vi "4461.Create.Sample Clock.vi"(8 "error in (no error)":errorcluster, 11 "LockinDAQ":refnum<class "LockinDAQ.lvclass">) -> (0 "error out":errorcluster, 3 "LockinDAQ out":refnum<class "LockinDAQ.lvclass">)   [LabVIEW 2016, in "LockinDAQ.lvclass"]
uses:
  LockinDAQ.lvclass
  LockinDAQ.lvclass/LockinDAQ.ctl
  <vilib>/DAQmx/configure/timing.llb/DAQmx Timing (Sample Clock).vi
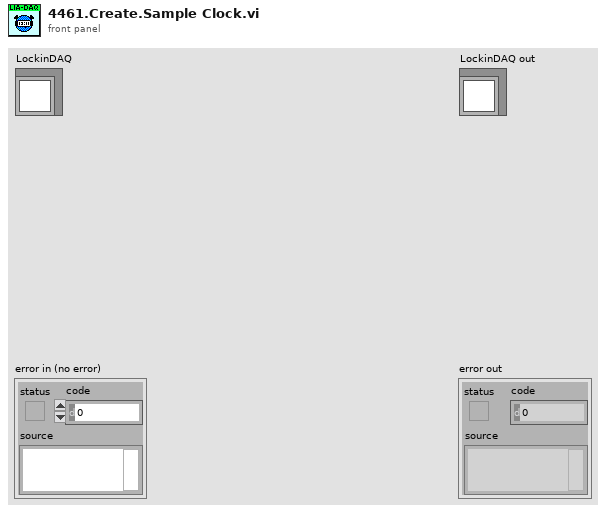
[diagram p1: front panel]
types:
  T1 = typedef "LockinDAQ.lvclass/DAQType-enum.ctl" = enum16{"None", "USB 4431", "PXI 446x"}
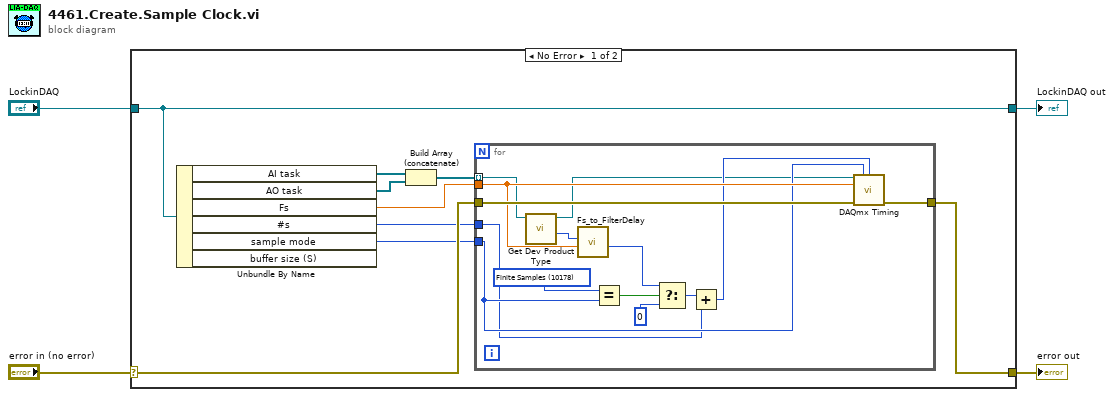
[diagram p0: block diagram]
diagram:
  n1 = case shown="No Error" "error in (no error)" {
    selector: "error in (no error)" -> [w7 w29]
    tunnel: [w8 w29] -> w3
    tunnel: [w13 w28] -> w1
    tunnel: "LockinDAQ" -> [w13 w28]
    frame No Error {
      n2 = Unbundle By Name(w13) -> ("AI task"=w12:refnum<k21>[], "AO task"=w11:refnum<k21>[], "Fs"=w9:dbl, "#s"=w5:i32, "sample mode"=w6:i32)  [unwired: 1 out]
      n3 = Build Array (concatenate)(w12, w11) -> (w10:refnum<k21>[])
      n4 = for {
        tunnel: w10 -> [w16] mode=indexing
        tunnel: w9 -> [w24]
        tunnel: w7 -> [w27]
        tunnel: [w26] -> w8
        tunnel: w6 -> [w17]
        tunnel: w5 -> [w14]
        w20 = 10178 items=["Finite Samples"=10178, "Continuous Samples"=10123] ("sample mode 2")
        n5 = call "Get Dev Product Type.vi"("Refnum in"=w16) -> ("DAQ Type"=w25:T1, "Refnum out"=w15:refnum<k21>)  [unwired: 7 in, 2 out]
        n6 = call "Fs_to_FilterDelay.vi"("Fs"=w24, "DAQ Type"=w25) -> ("Total Filter Delay (samples)"=w19:u32)  [unwired: 9 in]
        n7 = Equal?(x=w20, y=w17) -> (x = y?=w21:bool)
        n8 = Select(t=w19, s=w21, f=0) -> (s? t:f=w22:u32)
        n9 = Add(x=w22, y=w14) -> (x+y=w18:u32)
        n10 = call-poly <vilib>:"DAQmx Timing.vi"("task/channels in"=w15, "sample mode"=w17, "samples per channel"=w18, "rate"=w24, "error in"=w27) -> ("error out"=w26:errorcluster)  [unwired: 9 in, 1 out]
      }
    }
    frame Error {
    }
  }
  "error out" <- w3
  "LockinDAQ out" <- w1
